vi "GT_crdSpace.vi"(9 "fifo":i16, 10 "crd":i16, 11 "rtn_In":cluster{"rtn":i16, "Func":string}) -> (0 "fifo out":i16, 1 "pSpace":i32, 2 "crd out":i16, 3 "rtn_Out":cluster{"rtn":i16, "Func":string})   [LabVIEW 2014]
uses:
  VC6/gts.dll
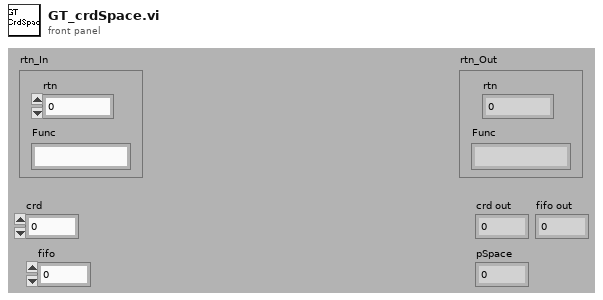
[diagram p1: front panel]
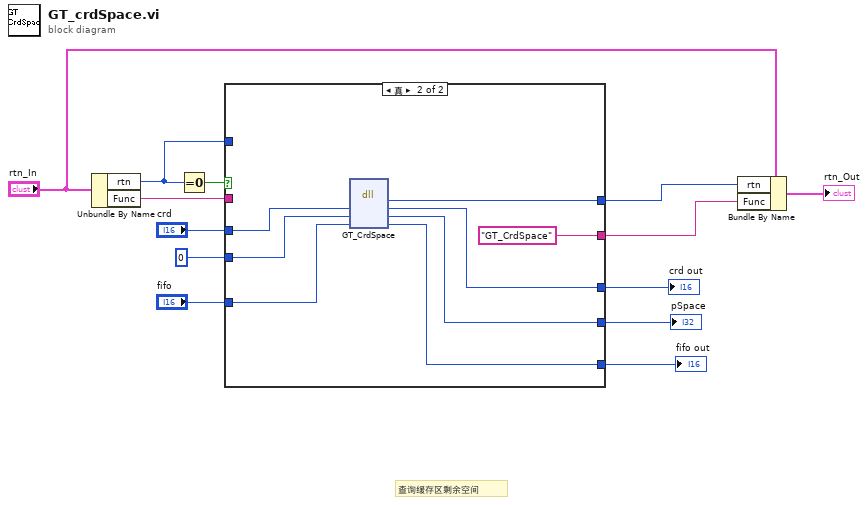
[diagram p0: block diagram]
diagram:
  # "查询缓存区剩余空间"
  n1 = Unbundle By Name("rtn_In") -> ("rtn"=w8:i16, "Func"=w7:string)
  n2 = Equal To 0?(x=w8) -> (x = 0?=w13:bool)
  n3 = case shown="真" w13 {
    tunnel: [w18 w26] -> w10
    tunnel: [w17 "GT_CrdSpace" ("Func")] -> w9
    tunnel: w8 -> [w18 _]
    tunnel: w7 -> [w17 _]
    tunnel: "crd" -> [w16 w24]
    tunnel: 0 ("pSpace") -> [w14 w23]
    tunnel: "fifo" -> [w15 w22]
    tunnel: [w16 w21] -> w3
    tunnel: [w14 w20] -> w2
    tunnel: [w15 w19] -> w1
    frame False {
    }
    frame True {
      n4 = dll-call lib="PTH2Fabs DNewGTS AC-800LWin7版源程序-20170926gts85VC6gts.dll" fn="GT_CrdSpace"("crd"=w24, "pSpace"=w23, "fifo"=w22) -> ("rtn"=w26:i16, "crd"=w21:i16, "pSpace"=w20:i32, "fifo"=w19:i16)  [unwired: 3 in, 2 out]
    }
  }
  "crd out" <- w3
  "pSpace" <- w2
  "fifo out" <- w1
  n5 = Bundle By Name(cluster="rtn_In", "rtn"=w10, "Func"=w9) -> (→"rtn_Out":cluster{"rtn":i16, "Func":string})
